vi "Main_UI.vi"(0 "ADC Type":T1, 1 "Edit":bool, 2 "Start":bool, 5 "No. of Bits":u8=1 min=1 max=16, 7 "No. of Channels":u8=1 min=1 max=8, 9 "Sampling Rate(ms)":u8=50 min=50, 11 "Error in":errorcluster, 12 "Confirm":bool, 13 "File Path":path=path "C:/Users/sadhana.suresh/Documents/SVN_Practice/SDLC/Sadhana/SUBMISSION D/Files/Data.txt", 14 "OK Btn":bool) -> (4 "Digital Waveform Graph":digitaldata(graph), 15 "Error out":errorcluster)   [LabVIEW 2020, in "ADC_MultiChannel.lvlib"]
doc: "This the GUI VI. It has a Home page, ADCs Available page and Instructions page. The Instructions are displayed in the Instructions page. The ADCs available with its configuration is displayed in the ADCs Available page. The Home page has all the controls and indicators for the main functionality. Here the ADC can be chosen and its specifications are displayed. When START is pressed the data acquisition starts and the digital data is plotted. Individual channels can be chosen to view them. By pressing EDIT CONFIGURATION the current ADC's specifications can be editted. Panel close will STOP the VI running."
uses:
  ADC_MultiChannel.lvlib
  Typedefs/ADC_Types.ctl
  Typedefs/Queue_Operations.ctl
  Typedefs/Data_Cluster_ip.ctl
  <vilib>/Utility/config.llb/Write Key (I32).vi
  <vilib>/Utility/config.llb/Read Key (I32).vi
  <vilib>/Utility/file.llb/Write Delimited Spreadsheet (I64).vi
  <vilib>/Utility/config.llb/NI_LVConfig.lvlib
panel:
  in  "Tab Control":enum32{"Home", "ADCs Available", "Instructions"}(tab)
  out "Sampling Rate":i32
  out "Channels":i32
  out "Bits":i32
  in  "Channel 1":bool
  in  "Channel 2":bool
  in  "Channel 3":bool
  in  "Channel 4":bool
  in  "Channel 5":bool
  in  "Channel 6":bool
  in  "Channel 7":bool
  in  "Channel 8":bool
  out "Message":string
  in  "Back Btn":bool
  out "Details":string
  out "Instructions":string
  # "ADC"
  # "CHANNEL"
  # "No. of Bits"
  # "No. of Channels"
  # "Sampling Rate"
  # "SELECTOR"
  # "MULTICHANNEL ADC"
  # "SOLITON"
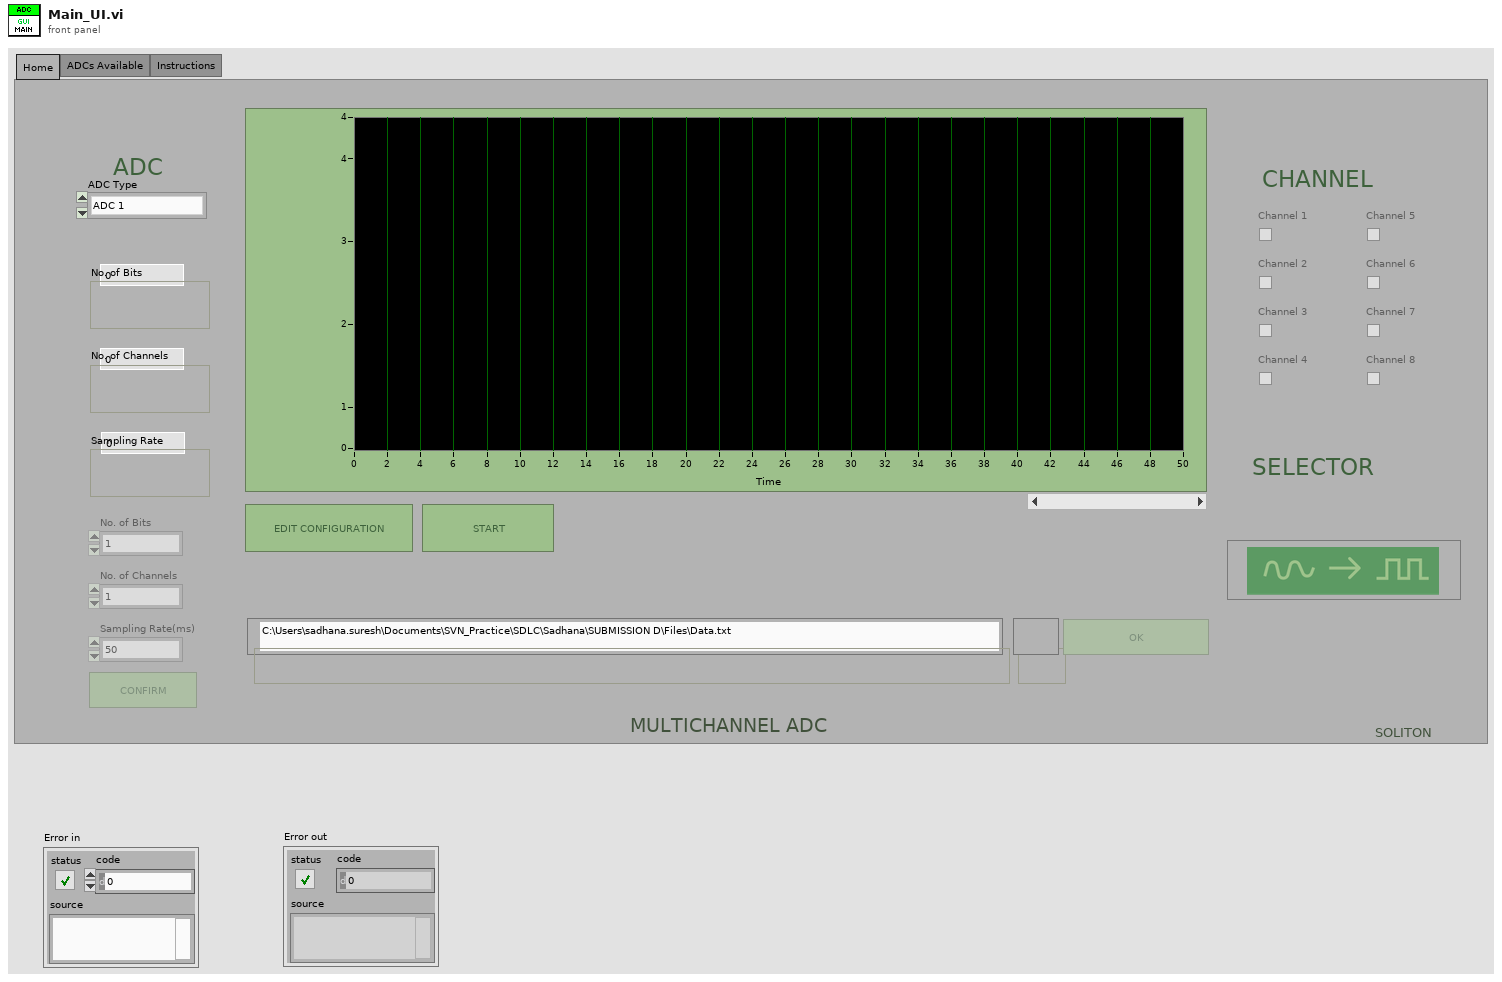
[diagram p1: front panel]
types:
  T1 = typedef "ADC_MultiChannel.lvlib/ADC_Types.ctl" = enum16{"ADC 1", "ADC 2", "ADC 3"}
  T2 = typedef "ADC_MultiChannel.lvlib/Data_Cluster_ip.ctl" = cluster{"ADC Type":string, "Bits":i32, "Channels":i32, "Sampling Rate":i32, "Digital Data":u8[][], "Start":bool, "File Path":path, "Analog Data":dbl[], "Channels ON":bool[], "OK Btn":bool, "Message":string, "Changed Channels":u8, "Changed Bits":u8, "Changed Rate":u8, "ADC Config File":path, "Edit":bool}
  T3 = typedef "ADC_MultiChannel.lvlib/Queue_Operations.ctl" = enum16{"Create Queue", "Enqueue element", "Dequeue", "Flush Queue", "Close Queue"}
  T4 = enum8{"Enabled", "Disabled", "Disabled and Grayed Out"}
  T5 = enum16{"open", "replace", "create", "open or create", "replace or create", "replace or create with confirmation"}
  T6 = typedef "NI_LVConfig.lvlib/Config Data RefNum.ctl" = refnum<k1>
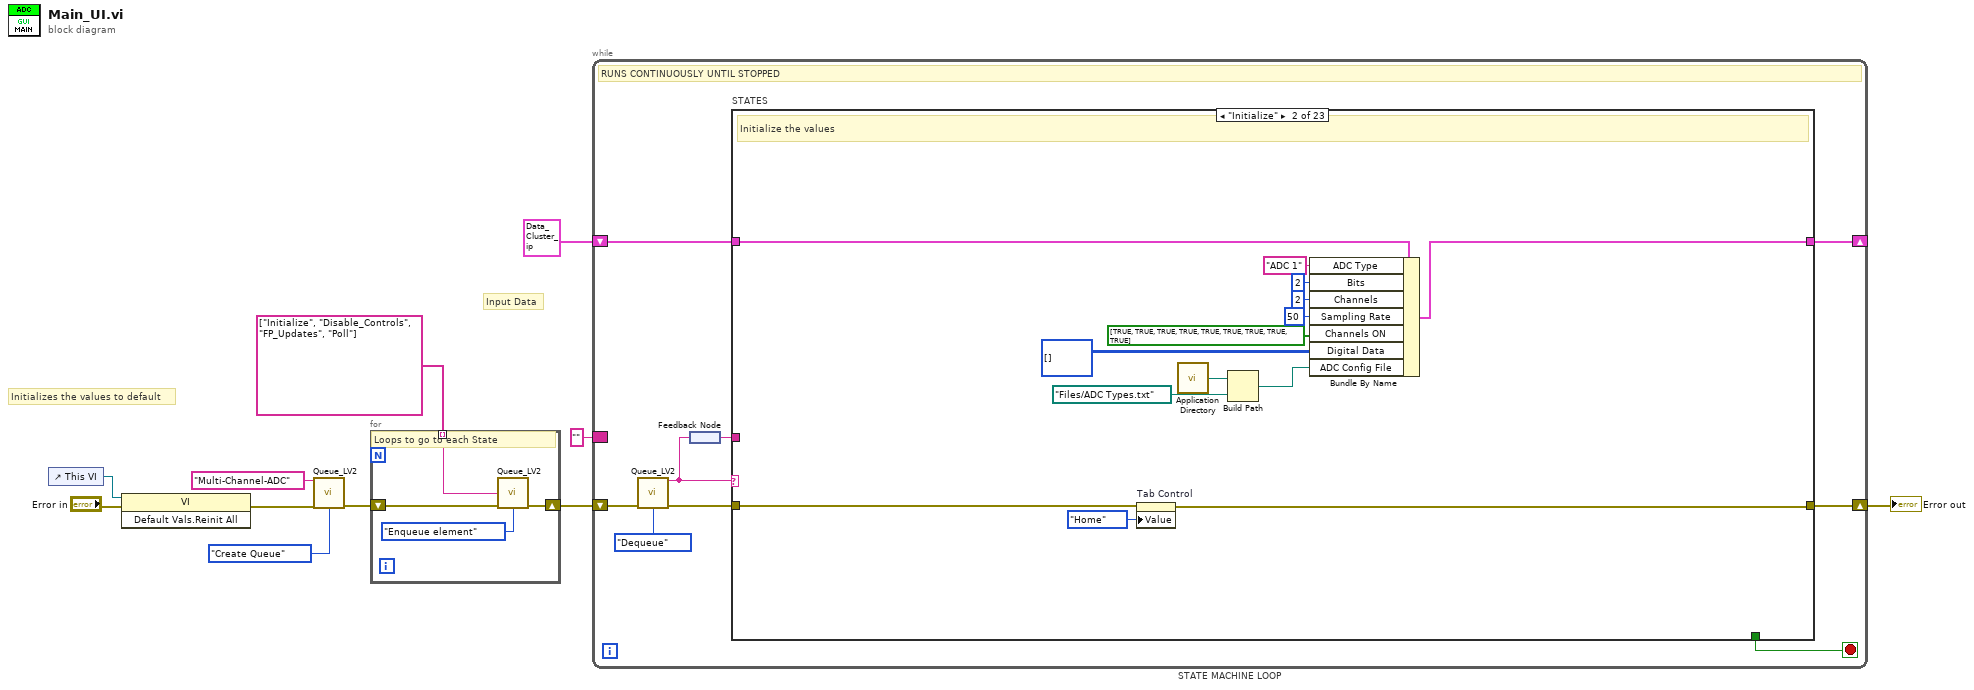
[diagram p0: block diagram]
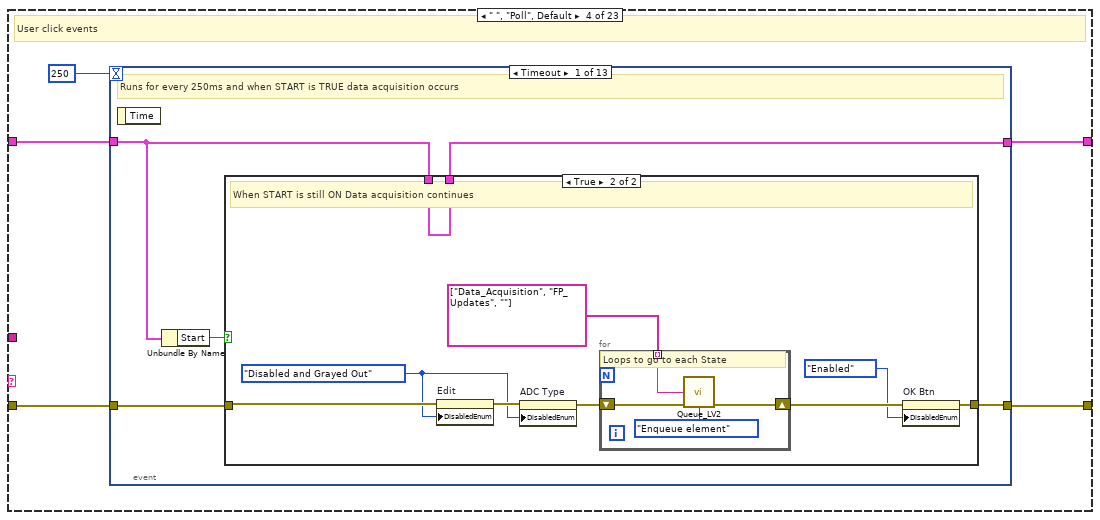
[diagram p4: hidden frame]
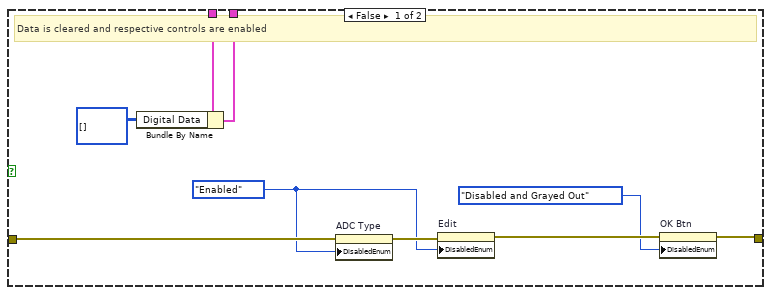
[diagram p5: hidden frame]
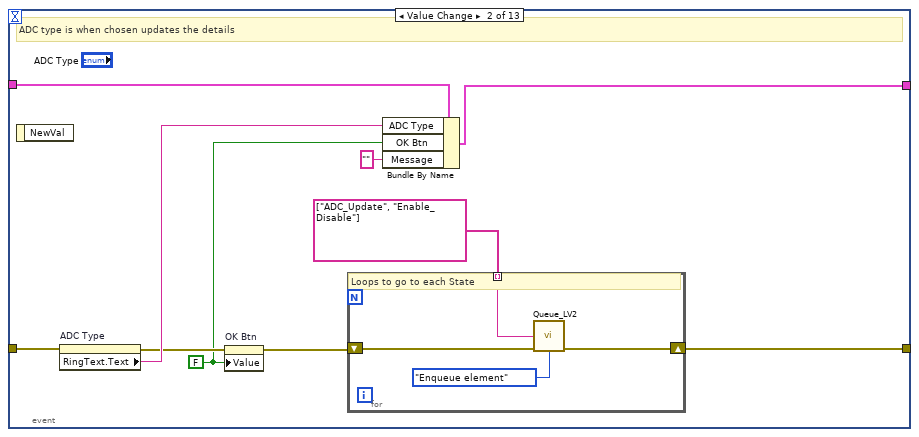
[diagram p6: hidden frame]
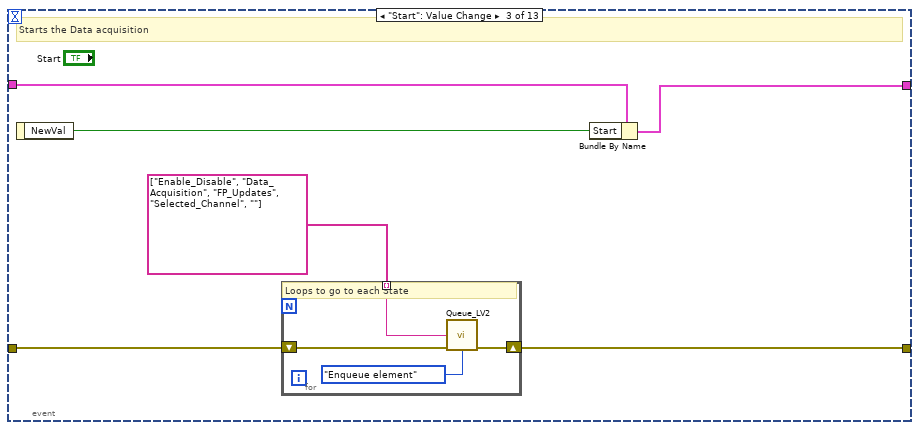
[diagram p7: hidden frame]
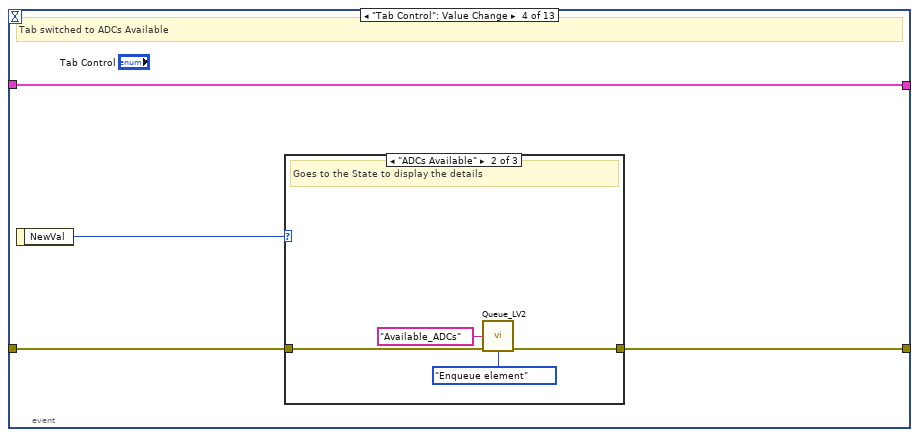
[diagram p8: hidden frame]
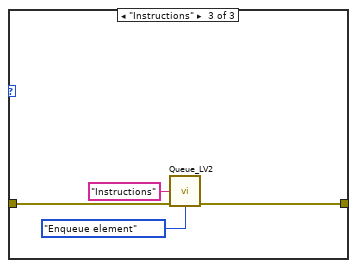
[diagram p10: hidden frame]
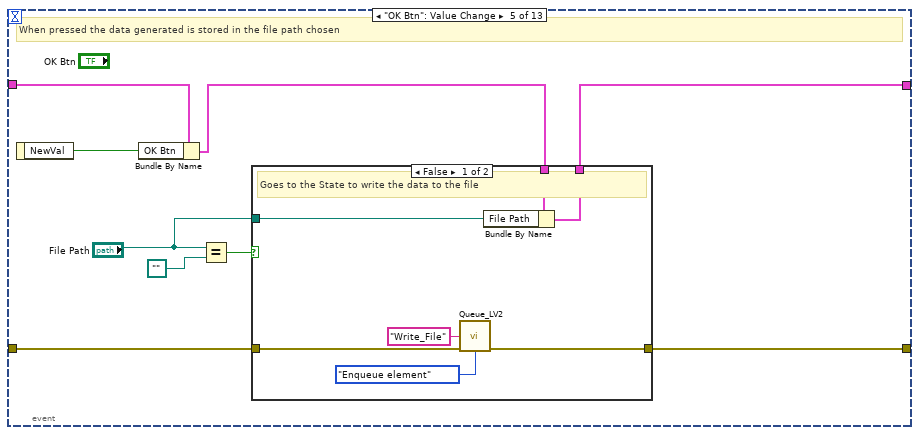
[diagram p11: hidden frame]
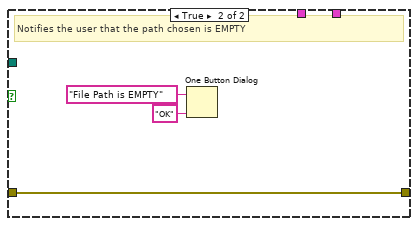
[diagram p12: hidden frame]
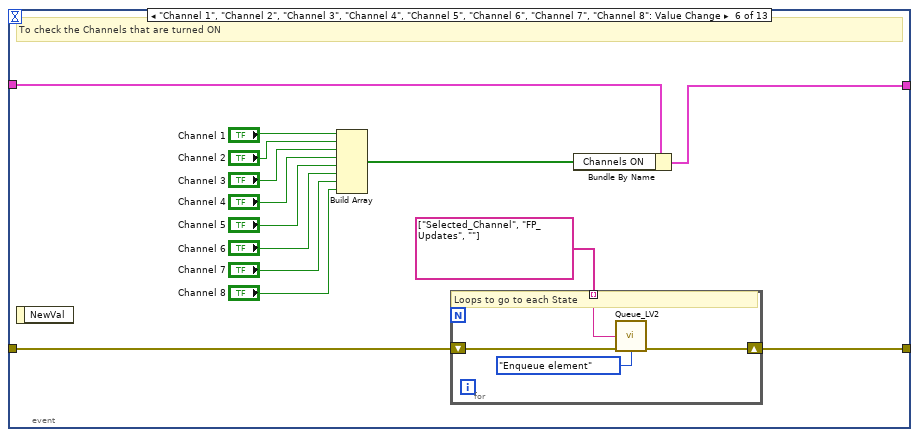
[diagram p13: hidden frame]
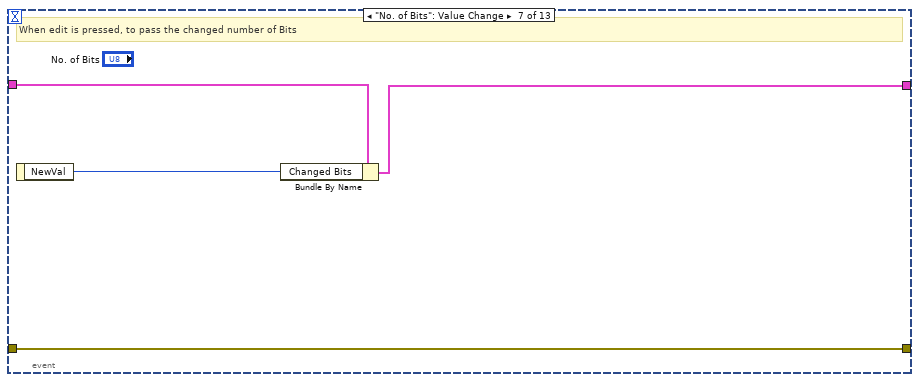
[diagram p14: hidden frame]
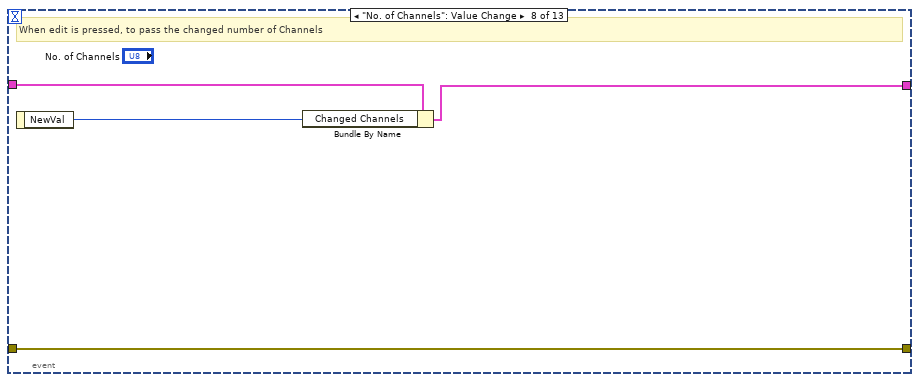
[diagram p15: hidden frame]
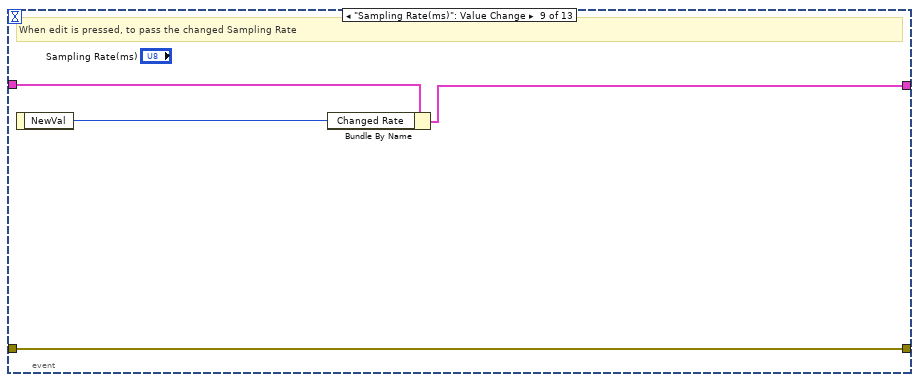
[diagram p16: hidden frame]
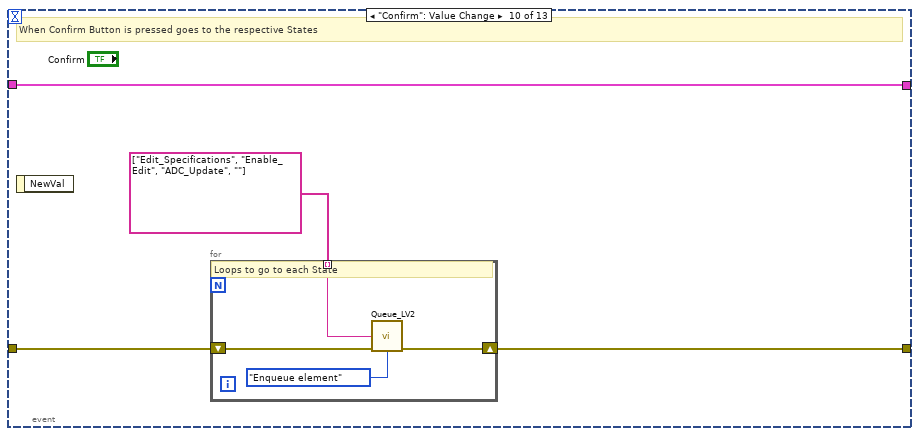
[diagram p17: hidden frame]
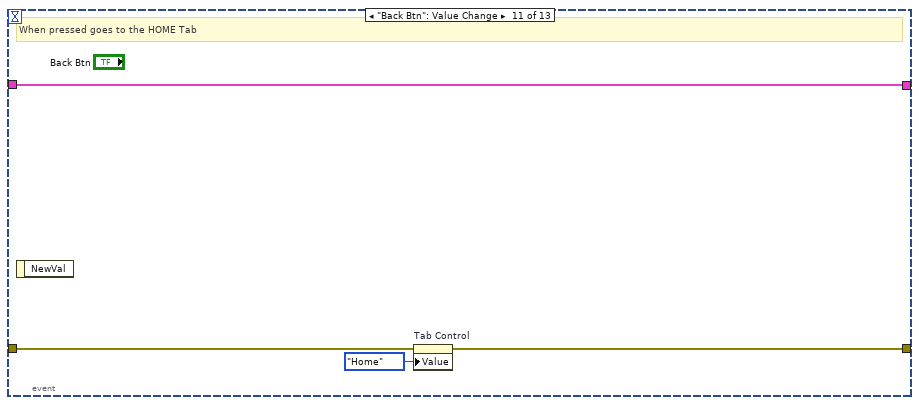
[diagram p18: hidden frame]
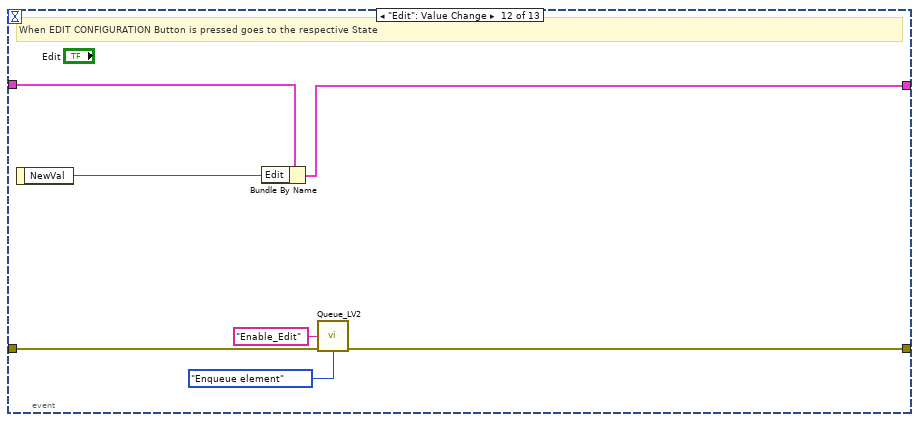
[diagram p19: hidden frame]
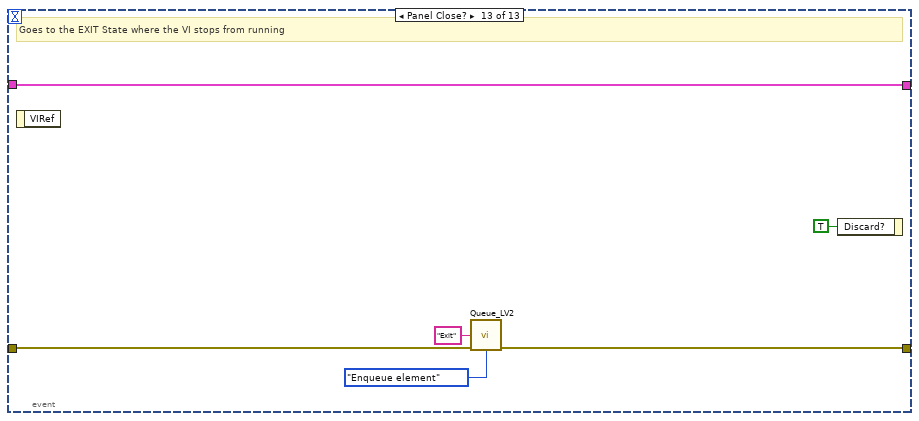
[diagram p20: hidden frame]
diagram:
  # "Input Data"
  # "Initializes the values to default"
  n1 = control-ref of="This VI"() -> (w4:refnum<vi>)
  n2 = invoke class="VI" method="Default Vals.Reinit All"(reference=w4, error in="Error in") -> (error out=w2:errorcluster)  [unwired: 1 in, 2 out]
  n3 = call "Queue_LV2.vi"("Name"="Multi-Channel-ADC", "Error in"=w2, "Queue Operations"=Queue_Operations."Create Queue") -> ("Error out"=w10:errorcluster)  [unwired: 11 in, 1 out]
  n4 = for {
    shift-right: [w14] -> w9
    shift-left: w10 -> [w15]
    tunnel: string[] ["Initialize", "Disable_Controls", "FP_Updates", "Poll"] -> [w12] mode=indexing
    # "Loops to go to each State"
    n5 = call "Queue_LV2.vi"("State"=w12, "Error in"=w15, "Queue Operations"=Queue_Operations."Enqueue element") -> ("Error out"=w14:errorcluster)  [unwired: 11 in, 1 out]
  }
  n6 = while "STATE MACHINE LOOP" {
    shift-right: [w19] -> _
    shift-left: T2 {"ADC Type"="", "Bits"=0, "Channels"=0, "Sampling Rate"=0, "Digital Data"=[], "Start"=FALSE, "File Path"=path "", "Analog Data"=[], "Channels ON"=[], "OK Btn"=FALSE, "Message"="", "Changed Channels"=1, "Changed Bits"=1, "Changed Rate"=50, "ADC Config File"=path "", "Edit"=FALSE} -> [w20]
    shift-right: [w21] -> w6
    shift-left: w9 -> [w24]
    border: "" ("Dequeue State") -> [_]
    stop <- w18 stop-if-true
    # "RUNS CONTINUOUSLY UNTIL STOPPED"
    n7 = call "Queue_LV2.vi"("Error in"=w24, "Queue Operations"=Queue_Operations."Dequeue") -> ("Dequeue State"=w17:string, "Error out"=w22:errorcluster)  [unwired: 12 in]
    n8 = feedback-in #1(w17) -> ()
    n9 = feedback #1() -> (w16:string)
    n10 = case "STATES" shown="\"Initialize\"" w17 {
      tunnel: w22 -> [w25 w28 w41 w44 w187 w191 w205 w344 w361 w363 w372 w399 w412 w439 w454 w489 w496 w503 w516 w520 w526 w529 w543]
      tunnel: [w25 w32 w41 w43 w187 w192 w204 w343 w361 w363 w372 w379 w403 w428 w453 w479 w496 w501 w508 w520 w524 w529 w531] -> w21
      tunnel: w20 -> [w26 w40 w42 w46 w188 w203 w207 w342 w362 w368 w373 w376 w409 w433 w455 w484 w497 w499 w519 w521 w528 w530 w534]
      tunnel: [w26 w35 w42 w45 w188 w203 w207 w342 w362 w368 w373 w375 w408 w426 w455 w482 w497 w499 w519 w521 w528 w530 w534] -> w19
      tunnel: [_ _ _ _ _ _ _ _ _ _ _ _ _ _ _ _ _ _ _ _ TRUE _ _] -> w18
      tunnel: w16 -> [_ _ _ _ _ _ _ _ _ _ _ _ _ _ _ _ _ _ _ _ _ _ w541]
      frame "<---------------------Initialize--------------------->" {
        # "Splitter Case"
      }
      frame "Initialize" {
        # "Initialize the values"
        n11 = property on="Tab Control" class="TabCtl (strict)"(error in=w28, "Value"=enum32{"Home", "ADCs Available", "Instructions"}."Home" ("Tab Control")) -> (error out=w32:errorcluster)  [unwired: 1 in, 1 out]
        n12 = call <vilib>:"Application Directory.vi"() -> ("Application Directory"=w31:path)
        n13 = Build Path(base path=w31, name or relative path=path "Files/ADC Types.txt") -> (appended path=w29:path)
        n14 = Bundle By Name(cluster=w40, "ADC Type"="ADC 1", "Bits"=2, "Channels"=2, "Sampling Rate"=50, "Channels ON"=bool[] [TRUE, TRUE, TRUE, TRUE, TRUE, TRUE, TRUE, TRUE, TRUE], "Digital Data"=u8[][] [], "ADC Config File"=w29) -> (w35:T2)
      }
      frame "<-------------User Click Event--------------->" {
        # "Splitter Case"
      }
      frame " ", "Poll", Default {
        # "User click events"
        n15 = event shown="[0] Timeout" {
          selector: _ -> [_ _ _ _ _ _ _ _ _ _ _ _ _]
          dyn-events: _ -> [_ _ _ _ _ _ _ _ _ _ _ _ _]
          timeout: 250 -> [_ _ _ _ _ _ _ _ _ _ _ _ _]
          tunnel: w46 -> [w49 w84 w91 w102 w114 w137 w151 w157 w161 w165 w173 w176 w186]
          tunnel: [w48 w83 w90 w102 w116 w135 w150 w155 w159 w165 w173 w175 w186] -> w45
          tunnel: w44 -> [w51 w82 w94 w101 w118 w134 w153 w154 w158 w164 w172 w180 w185]
          tunnel: [w50 w76 w93 w100 w117 w133 w153 w154 w158 w163 w171 w179 w184] -> w43
          event Timeout {
            # "Runs for every 250ms and when START is TRUE data acquisition occurs"
            n16 = event-data() -> ()  [unwired: 1 in, 1 out]
            n17 = Unbundle By Name(w49) -> ("Start"=w52:bool)
            n18 = case shown="True" w52 {
              tunnel: w51 -> [w61 w65]
              tunnel: [w54 w63] -> w50
              tunnel: w49 -> [w60 w67]
              tunnel: [w59 w67] -> w48
              frame False {
                w55 = T4."Enabled" ("Disabled")
                # "Data is cleared and respective controls are enabled"
                n19 = Bundle By Name(cluster=w60, "Digital Data"=u8[][] []) -> (w59:T2)
                n20 = property on="ADC Type" class="Enum (strict)"(error in=w61, "DisabledEnum"=w55) -> (error out=w57:errorcluster)  [unwired: 1 in, 1 out]
                n21 = property on="Edit" class="Bool (strict)"(error in=w57, "DisabledEnum"=w55) -> (error out=w56:errorcluster)  [unwired: 1 in, 1 out]
                n22 = property on="OK Btn" class="Bool (strict)"(error in=w56, "DisabledEnum"=T4."Disabled and Grayed Out" ("Disabled")) -> (error out=w54:errorcluster)  [unwired: 1 in, 1 out]
              }
              frame True {
                w64 = T4."Disabled and Grayed Out" ("Disabled")
                # "When START is still ON Data acquisition continues"
                n23 = property on="Edit" class="Bool (strict)"(error in=w65, "DisabledEnum"=w64) -> (error out=w66:errorcluster)  [unwired: 1 in, 1 out]
                n24 = property on="ADC Type" class="Enum (strict)"(error in=w66, "DisabledEnum"=w64) -> (error out=w68:errorcluster)  [unwired: 1 in, 1 out]
                n25 = for {
                  shift-right: [w73] -> w70
                  shift-left: w68 -> [w74]
                  tunnel: string[] ["Data_Acquisition", "FP_Updates", ""] -> [w71] mode=indexing
                  # "Loops to go to each State"
                  n26 = call "Queue_LV2.vi"("State"=w71, "Error in"=w74, "Queue Operations"=Queue_Operations."Enqueue element") -> ("Error out"=w73:errorcluster)  [unwired: 11 in, 1 out]
                }
                n27 = property on="OK Btn" class="Bool (strict)"(error in=w70, "DisabledEnum"=T4."Enabled" ("Disabled")) -> (error out=w63:errorcluster)  [unwired: 1 in, 1 out]
              }
            }
          }
          event Value Change {
            w77 = FALSE ("OK Btn")
            # "ADC type is when chosen updates the details"
            n28 = event-data() -> ()  [unwired: 1 in, 1 out]
            n29 = property on="ADC Type" class="Enum (strict)"(error in=w82) -> (error out=w78:errorcluster, "RingText.Text"=w81:string)  [unwired: 1 in, 1 out]
            n30 = property on="OK Btn" class="Bool (strict)"(error in=w78, "Value"=w77) -> (error out=w79:errorcluster)  [unwired: 1 in, 1 out]
            n31 = for {
              shift-right: [w87] -> w76
              shift-left: w79 -> [w88]
              tunnel: string[] ["ADC_Update", "Enable_Disable"] -> [w85] mode=indexing
              # "Loops to go to each State"
              n32 = call "Queue_LV2.vi"("State"=w85, "Error in"=w88, "Queue Operations"=Queue_Operations."Enqueue element") -> ("Error out"=w87:errorcluster)  [unwired: 11 in, 1 out]
            }
            n33 = Bundle By Name(cluster=w84, "ADC Type"=w81, "OK Btn"=w77, "Message"="") -> (w83:T2)
          }
          event "Start": Value Change {
            # "Starts the Data acquisition"
            n34 = event-data() -> ("NewVal"=w89:bool)  [unwired: 1 in]
            n35 = for {
              shift-right: [w97] -> w93
              shift-left: w94 -> [w98]
              tunnel: string[] ["Enable_Disable", "Data_Acquisition", "FP_Updates", "Selected_Channel", ""] -> [w95] mode=indexing
              # "Loops to go to each State"
              n36 = call "Queue_LV2.vi"("State"=w95, "Error in"=w98, "Queue Operations"=Queue_Operations."Enqueue element") -> ("Error out"=w97:errorcluster)  [unwired: 11 in, 1 out]
            }
            n37 = Bundle By Name(cluster=w91, "Start"=w89) -> (w90:T2)
          }
          event "Tab Control": Value Change {
            # "Tab switched to ADCs Available"
            n38 = event-data() -> ("NewVal"=w99:enum32{"Home", "ADCs Available", "Instructions"})  [unwired: 1 in]
            n39 = case shown="\"ADCs Available\"" w99 {
              tunnel: w101 -> [w103 w106 w111]
              tunnel: [w103 w105 w110] -> w100
              frame "Home", Default {
                # "Nothing Happens"
              }
              frame "ADCs Available" {
                # "Goes to the State to display the details"
                n40 = call "Queue_LV2.vi"("State"="Available_ADCs", "Error in"=w106, "Queue Operations"=Queue_Operations."Enqueue element") -> ("Error out"=w105:errorcluster)  [unwired: 11 in, 1 out]
              }
              frame "Instructions" {
                n41 = call "Queue_LV2.vi"("State"="Instructions", "Error in"=w111, "Queue Operations"=Queue_Operations."Enqueue element") -> ("Error out"=w110:errorcluster)  [unwired: 11 in, 1 out]
              }
            }
          }
          event "OK Btn": Value Change {
            # "When pressed the data generated is stored in the file path chosen"
            n42 = event-data() -> ("NewVal"=w112:bool)  [unwired: 1 in]
            n43 = Bundle By Name(cluster=w114, "OK Btn"=w112) -> (w113:T2)
            n44 = Equal?(x="File Path", y=path "") -> (x = y?=w119:bool)
            n45 = case shown="False" w119 {
              tunnel: w118 -> [w124 w129]
              tunnel: [w123 w129] -> w117
              tunnel: w113 -> [w127 w128]
              tunnel: [w126 w128] -> w116
              tunnel: "File Path" -> [w125 _]
              frame False {
                # "Goes to the State to write the data to the file"
                n46 = call "Queue_LV2.vi"("State"="Write_File", "Error in"=w124, "Queue Operations"=Queue_Operations."Enqueue element") -> ("Error out"=w123:errorcluster)  [unwired: 11 in, 1 out]
                n47 = Bundle By Name(cluster=w127, "File Path"=w125) -> (w126:T2)
              }
              frame True {
                # "Notifies the user that the path chosen is EMPTY"
                n48 = One Button Dialog(message="File Path is EMPTY", button name ("OK")="OK") -> ()  [unwired: 1 out]
              }
            }
          }
          event "Channel 1", "Channel 2", "Channel 3", "Channel 4", "Channel 5", "Channel 6", "Channel 7", "Channel 8": Value Change {
            # "To check the Channels that are turned ON"
            n49 = event-data() -> ()  [unwired: 1 in, 1 out]
            n50 = Build Array("Channel 1", "Channel 2", "Channel 3", "Channel 4", "Channel 5", "Channel 6", "Channel 7", "Channel 8") -> (w136:bool[])
            n51 = for {
              shift-right: [w148] -> w133
              shift-left: w134 -> [w149]
              tunnel: string[] ["Selected_Channel", "FP_Updates", ""] -> [w146] mode=indexing
              # "Loops to go to each State"
              n52 = call "Queue_LV2.vi"("State"=w146, "Error in"=w149, "Queue Operations"=Queue_Operations."Enqueue element") -> ("Error out"=w148:errorcluster)  [unwired: 11 in, 1 out]
            }
            n53 = Bundle By Name(cluster=w137, "Channels ON"=w136) -> (w135:T2)
          }
          event "No. of Bits": Value Change {
            # "When edit is pressed, to pass the changed number of Bits"
            n54 = event-data() -> ("NewVal"=w152:u8)  [unwired: 1 in]
            n55 = Bundle By Name(cluster=w151, "Changed Bits"=w152) -> (w150:T2)
          }
          event "No. of Channels": Value Change {
            # "When edit is pressed, to pass the changed number of Channels"
            n56 = event-data() -> ("NewVal"=w156:u8)  [unwired: 1 in]
            n57 = Bundle By Name(cluster=w157, "Changed Channels"=w156) -> (w155:T2)
          }
          event "Sampling Rate(ms)": Value Change {
            # "When edit is pressed, to pass the changed Sampling Rate"
            n58 = event-data() -> ("NewVal"=w160:u8)  [unwired: 1 in]
            n59 = Bundle By Name(cluster=w161, "Changed Rate"=w160) -> (w159:T2)
          }
          event "Confirm": Value Change {
            # "When Confirm Button is pressed goes to the respective States"
            n60 = event-data() -> ()  [unwired: 1 in, 1 out]
            n61 = for {
              shift-right: [w168] -> w163
              shift-left: w164 -> [w169]
              tunnel: string[] ["Edit_Specifications", "Enable_Edit", "ADC_Update", ""] -> [w166] mode=indexing
              # "Loops to go to each State"
              n62 = call "Queue_LV2.vi"("State"=w166, "Error in"=w169, "Queue Operations"=Queue_Operations."Enqueue element") -> ("Error out"=w168:errorcluster)  [unwired: 11 in, 1 out]
            }
          }
          event "Back Btn": Value Change {
            # "When pressed goes to the HOME Tab"
            n63 = event-data() -> ()  [unwired: 1 in, 1 out]
            n64 = property on="Tab Control" class="TabCtl (strict)"(error in=w172, "Value"=enum32{"Home", "ADCs Available", "Instructions"}."Home" ("Tab Control")) -> (error out=w171:errorcluster)  [unwired: 1 in, 1 out]
          }
          event "Edit": Value Change {
            # "When EDIT CONFIGURATION Button is pressed goes to the respective State"
            n65 = event-data() -> ("NewVal"=w174:bool)  [unwired: 1 in]
            n66 = Bundle By Name(cluster=w176, "Edit"=w174) -> (w175:T2)
            n67 = call "Queue_LV2.vi"("State"="Enable_Edit", "Error in"=w180, "Queue Operations"=Queue_Operations."Enqueue element") -> ("Error out"=w179:errorcluster)  [unwired: 11 in, 1 out]
          }
          event Panel Close? {
            # "Goes to the EXIT State where the VI stops from running"
            n68 = event-data() -> ()  [unwired: 1 in, 1 out]
            n69 = call "Queue_LV2.vi"("State"="Exit", "Error in"=w185, "Queue Operations"=Queue_Operations."Enqueue element") -> ("Error out"=w184:errorcluster)  [unwired: 11 in, 1 out]
            n70 = event-data("Discard?"=TRUE) -> ()  [unwired: 1 in, 1 out]
          }
        }
      }
      frame "<-----------------Enable and Disable---------------->" {
        # "Splitter Case"
      }
      frame "Disable_Controls" {
        w189 = T4."Disabled and Grayed Out" ("Disabled")
        # "Disable the Controls at the time of Initialization"
        n71 = property on="Confirm" class="Bool"(error in=w191, "DisabledEnum"=w189) -> (error out=w190:errorcluster)  [unwired: 1 in, 1 out]
        n72 = property on="Sampling Rate(ms)" class="DigNum (strict)"(error in=w190, "DisabledEnum"=w189) -> (error out=w193:errorcluster)  [unwired: 1 in, 1 out]
        n73 = property on="No. of Bits" class="DigNum (strict)"(error in=w193, "DisabledEnum"=w189) -> (error out=w195:errorcluster)  [unwired: 1 in, 1 out]
        n74 = property on="No. of Channels" class="DigNum (strict)"(error in=w195, "DisabledEnum"=w189) -> (error out=w194:errorcluster)  [unwired: 1 in, 1 out]
        n75 = property on="Channel 1" class="Bool (strict)"(error in=w194, "DisabledEnum"=w189) -> (error out=w202:errorcluster)  [unwired: 1 in, 1 out]
        n76 = property on="Channel 2" class="Bool (strict)"(error in=w202, "DisabledEnum"=w189) -> (error out=w201:errorcluster)  [unwired: 1 in, 1 out]
        n77 = property on="Channel 3" class="Bool (strict)"(error in=w201, "DisabledEnum"=w189) -> (error out=w200:errorcluster)  [unwired: 1 in, 1 out]
        n78 = property on="Channel 4" class="Bool (strict)"(error in=w200, "DisabledEnum"=w189) -> (error out=w199:errorcluster)  [unwired: 1 in, 1 out]
        n79 = property on="Channel 5" class="Bool (strict)"(error in=w199, "DisabledEnum"=w189) -> (error out=w198:errorcluster)  [unwired: 1 in, 1 out]
        n80 = property on="Channel 6" class="Bool (strict)"(error in=w198, "DisabledEnum"=w189) -> (error out=w197:errorcluster)  [unwired: 1 in, 1 out]
        n81 = property on="Channel 7" class="Bool (strict)"(error in=w197, "DisabledEnum"=w189) -> (error out=w196:errorcluster)  [unwired: 1 in, 1 out]
        n82 = property on="Channel 8" class="Bool (strict)"(error in=w196, "DisabledEnum"=w189) -> (error out=w192:errorcluster)  [unwired: 1 in, 1 out]
      }
      frame "Enable_Disable" {
        # "To Enable and Disable Channels according to the number of Channels present"
        n83 = Unbundle By Name(w207) -> ("Channels"=w206:i32)
        n84 = case shown="0, Default" w206 {
          tunnel: w205 -> [w217 w222 w235 w247 w262 w275 w292 w308 w325]
          tunnel: [w209 w221 w234 w246 w261 w276 w291 w309 w326] -> w204
          frame 0, Default {
            w208 = T4."Disabled and Grayed Out" ("Disabled")
            # "All the Channels are disabled"
            n85 = property on="Channel 1" class="Bool (strict)"(error in=w217, "DisabledEnum"=w208) -> (error out=w216:errorcluster)  [unwired: 1 in, 1 out]
            n86 = property on="Channel 2" class="Bool (strict)"(error in=w216, "DisabledEnum"=w208) -> (error out=w215:errorcluster)  [unwired: 1 in, 1 out]
            n87 = property on="Channel 3" class="Bool (strict)"(error in=w215, "DisabledEnum"=w208) -> (error out=w214:errorcluster)  [unwired: 1 in, 1 out]
            n88 = property on="Channel 4" class="Bool (strict)"(error in=w214, "DisabledEnum"=w208) -> (error out=w213:errorcluster)  [unwired: 1 in, 1 out]
            n89 = property on="Channel 5" class="Bool (strict)"(error in=w213, "DisabledEnum"=w208) -> (error out=w212:errorcluster)  [unwired: 1 in, 1 out]
            n90 = property on="Channel 6" class="Bool (strict)"(error in=w212, "DisabledEnum"=w208) -> (error out=w211:errorcluster)  [unwired: 1 in, 1 out]
            n91 = property on="Channel 7" class="Bool (strict)"(error in=w211, "DisabledEnum"=w208) -> (error out=w210:errorcluster)  [unwired: 1 in, 1 out]
            n92 = property on="Channel 8" class="Bool (strict)"(error in=w210, "DisabledEnum"=w208) -> (error out=w209:errorcluster)  [unwired: 1 in, 1 out]
          }
          frame 1 {
            w219 = T4."Disabled and Grayed Out" ("Disabled")
            # "When the total number of Channel is 1 the 1st channel alone is enabled"
            n93 = property on="Channel 1" class="Bool (strict)"(error in=w222, "DisabledEnum"=T4."Enabled" ("Disabled"), "Value"=TRUE ("Channel 1")) -> (error out=w229:errorcluster)  [unwired: 1 in, 1 out]
            n94 = property on="Channel 2" class="Bool (strict)"(error in=w229, "DisabledEnum"=w219) -> (error out=w228:errorcluster)  [unwired: 1 in, 1 out]
            n95 = property on="Channel 3" class="Bool (strict)"(error in=w228, "DisabledEnum"=w219) -> (error out=w227:errorcluster)  [unwired: 1 in, 1 out]
            n96 = property on="Channel 4" class="Bool (strict)"(error in=w227, "DisabledEnum"=w219) -> (error out=w226:errorcluster)  [unwired: 1 in, 1 out]
            n97 = property on="Channel 5" class="Bool (strict)"(error in=w226, "DisabledEnum"=w219) -> (error out=w225:errorcluster)  [unwired: 1 in, 1 out]
            n98 = property on="Channel 6" class="Bool (strict)"(error in=w225, "DisabledEnum"=w219) -> (error out=w224:errorcluster)  [unwired: 1 in, 1 out]
            n99 = property on="Channel 7" class="Bool (strict)"(error in=w224, "DisabledEnum"=w219) -> (error out=w223:errorcluster)  [unwired: 1 in, 1 out]
            n100 = property on="Channel 8" class="Bool (strict)"(error in=w223, "DisabledEnum"=w219) -> (error out=w221:errorcluster)  [unwired: 1 in, 1 out]
          }
          frame 2 {
            w232 = T4."Disabled and Grayed Out" ("Disabled")
            w233 = T4."Enabled" ("Disabled")
            # "When the total number of Channels are 2 the 1st and 2nd channels alone are enabled"
            n101 = property on="Channel 1" class="Bool (strict)"(error in=w235, "DisabledEnum"=w233, "Value"=TRUE ("Channel 1")) -> (error out=w242:errorcluster)  [unwired: 1 in, 1 out]
            n102 = property on="Channel 2" class="Bool (strict)"(error in=w242, "DisabledEnum"=w233, "Value"=TRUE ("Channel 2")) -> (error out=w241:errorcluster)  [unwired: 1 in, 1 out]
            n103 = property on="Channel 3" class="Bool (strict)"(error in=w241, "DisabledEnum"=w232) -> (error out=w240:errorcluster)  [unwired: 1 in, 1 out]
            n104 = property on="Channel 4" class="Bool (strict)"(error in=w240, "DisabledEnum"=w232) -> (error out=w239:errorcluster)  [unwired: 1 in, 1 out]
            n105 = property on="Channel 5" class="Bool (strict)"(error in=w239, "DisabledEnum"=w232) -> (error out=w238:errorcluster)  [unwired: 1 in, 1 out]
            n106 = property on="Channel 6" class="Bool (strict)"(error in=w238, "DisabledEnum"=w232) -> (error out=w237:errorcluster)  [unwired: 1 in, 1 out]
            n107 = property on="Channel 7" class="Bool (strict)"(error in=w237, "DisabledEnum"=w232) -> (error out=w236:errorcluster)  [unwired: 1 in, 1 out]
            n108 = property on="Channel 8" class="Bool (strict)"(error in=w236, "DisabledEnum"=w232) -> (error out=w234:errorcluster)  [unwired: 1 in, 1 out]
          }
          frame 3 {
            w244 = T4."Disabled and Grayed Out" ("Disabled")
            w245 = T4."Enabled" ("Disabled")
            # "When the total number of Channels are 3 the 1st  2nd and 3rd channels alone are enabled"
            n109 = property on="Channel 1" class="Bool (strict)"(error in=w247, "DisabledEnum"=w245, "Value"=TRUE ("Channel 1")) -> (error out=w256:errorcluster)  [unwired: 1 in, 1 out]
            n110 = property on="Channel 2" class="Bool (strict)"(error in=w256, "DisabledEnum"=w245, "Value"=TRUE ("Channel 2")) -> (error out=w255:errorcluster)  [unwired: 1 in, 1 out]
            n111 = property on="Channel 3" class="Bool (strict)"(error in=w255, "DisabledEnum"=w245, "Value"=TRUE ("Channel 3")) -> (error out=w254:errorcluster)  [unwired: 1 in, 1 out]
            n112 = property on="Channel 4" class="Bool (strict)"(error in=w254, "DisabledEnum"=w244) -> (error out=w253:errorcluster)  [unwired: 1 in, 1 out]
            n113 = property on="Channel 5" class="Bool (strict)"(error in=w253, "DisabledEnum"=w244) -> (error out=w252:errorcluster)  [unwired: 1 in, 1 out]
            n114 = property on="Channel 6" class="Bool (strict)"(error in=w252, "DisabledEnum"=w244) -> (error out=w251:errorcluster)  [unwired: 1 in, 1 out]
            n115 = property on="Channel 7" class="Bool (strict)"(error in=w251, "DisabledEnum"=w244) -> (error out=w250:errorcluster)  [unwired: 1 in, 1 out]
            n116 = property on="Channel 8" class="Bool (strict)"(error in=w250, "DisabledEnum"=w244) -> (error out=w246:errorcluster)  [unwired: 1 in, 1 out]
          }
          frame 4 {
            w257 = T4."Disabled and Grayed Out" ("Disabled")
            w258 = T4."Enabled" ("Disabled")
            # "When the total number of Channels are 4 the 1st  2nd  3rd and 4th channels alone are enabled"
            n117 = property on="Channel 1" class="Bool (strict)"(error in=w262, "DisabledEnum"=w258, "Value"=TRUE ("Channel 1")) -> (error out=w271:errorcluster)  [unwired: 1 in, 1 out]
            n118 = property on="Channel 2" class="Bool (strict)"(error in=w271, "DisabledEnum"=w258, "Value"=TRUE ("Channel 2")) -> (error out=w270:errorcluster)  [unwired: 1 in, 1 out]
            n119 = property on="Channel 3" class="Bool (strict)"(error in=w270, "DisabledEnum"=w258, "Value"=TRUE ("Channel 3")) -> (error out=w269:errorcluster)  [unwired: 1 in, 1 out]
            n120 = property on="Channel 4" class="Bool (strict)"(error in=w269, "DisabledEnum"=w258, "Value"=TRUE ("Channel 4")) -> (error out=w268:errorcluster)  [unwired: 1 in, 1 out]
            n121 = property on="Channel 5" class="Bool (strict)"(error in=w268, "DisabledEnum"=w257) -> (error out=w267:errorcluster)  [unwired: 1 in, 1 out]
            n122 = property on="Channel 6" class="Bool (strict)"(error in=w267, "DisabledEnum"=w257) -> (error out=w266:errorcluster)  [unwired: 1 in, 1 out]
            n123 = property on="Channel 7" class="Bool (strict)"(error in=w266, "DisabledEnum"=w257) -> (error out=w265:errorcluster)  [unwired: 1 in, 1 out]
            n124 = property on="Channel 8" class="Bool (strict)"(error in=w265, "DisabledEnum"=w257) -> (error out=w261:errorcluster)  [unwired: 1 in, 1 out]
          }
          frame 5 {
            w272 = T4."Disabled and Grayed Out" ("Disabled")
            w274 = T4."Enabled" ("Disabled")
            # "When the total number of Channels are 5 the 1st  2nd  3rd 4th and 5th channels alone are enabled"
            n125 = property on="Channel 1" class="Bool (strict)"(error in=w275, "DisabledEnum"=w274, "Value"=TRUE ("Channel 1")) -> (error out=w287:errorcluster)  [unwired: 1 in, 1 out]
            n126 = property on="Channel 2" class="Bool (strict)"(error in=w287, "DisabledEnum"=w274, "Value"=TRUE ("Channel 2")) -> (error out=w286:errorcluster)  [unwired: 1 in, 1 out]
            n127 = property on="Channel 3" class="Bool (strict)"(error in=w286, "DisabledEnum"=w274, "Value"=TRUE ("Channel 3")) -> (error out=w285:errorcluster)  [unwired: 1 in, 1 out]
            n128 = property on="Channel 4" class="Bool (strict)"(error in=w285, "DisabledEnum"=w274, "Value"=TRUE ("Channel 4")) -> (error out=w284:errorcluster)  [unwired: 1 in, 1 out]
            n129 = property on="Channel 5" class="Bool (strict)"(error in=w284, "DisabledEnum"=w274, "Value"=TRUE ("Channel 5")) -> (error out=w283:errorcluster)  [unwired: 1 in, 1 out]
            n130 = property on="Channel 6" class="Bool (strict)"(error in=w283, "DisabledEnum"=w272) -> (error out=w282:errorcluster)  [unwired: 1 in, 1 out]
            n131 = property on="Channel 7" class="Bool (strict)"(error in=w282, "DisabledEnum"=w272) -> (error out=w281:errorcluster)  [unwired: 1 in, 1 out]
            n132 = property on="Channel 8" class="Bool (strict)"(error in=w281, "DisabledEnum"=w272) -> (error out=w276:errorcluster)  [unwired: 1 in, 1 out]
          }
          frame 6 {
            w288 = T4."Disabled and Grayed Out" ("Disabled")
            w290 = T4."Enabled" ("Disabled")
            # "When the total number of Channels are 6 the 1st  2nd  3rd 4th  5th and 6th channels alone are enabled"
            n133 = property on="Channel 1" class="Bool (strict)"(error in=w292, "DisabledEnum"=w290, "Value"=TRUE ("Channel 1")) -> (error out=w304:errorcluster)  [unwired: 1 in, 1 out]
            n134 = property on="Channel 2" class="Bool (strict)"(error in=w304, "DisabledEnum"=w290, "Value"=TRUE ("Channel 2")) -> (error out=w303:errorcluster)  [unwired: 1 in, 1 out]
            n135 = property on="Channel 3" class="Bool (strict)"(error in=w303, "DisabledEnum"=w290, "Value"=TRUE ("Channel 3")) -> (error out=w302:errorcluster)  [unwired: 1 in, 1 out]
            n136 = property on="Channel 4" class="Bool (strict)"(error in=w302, "DisabledEnum"=w290, "Value"=TRUE ("Channel 4")) -> (error out=w301:errorcluster)  [unwired: 1 in, 1 out]
            n137 = property on="Channel 5" class="Bool (strict)"(error in=w301, "DisabledEnum"=w290, "Value"=TRUE ("Channel 5")) -> (error out=w300:errorcluster)  [unwired: 1 in, 1 out]
            n138 = property on="Channel 6" class="Bool (strict)"(error in=w300, "DisabledEnum"=w290, "Value"=TRUE ("Channel 6")) -> (error out=w299:errorcluster)  [unwired: 1 in, 1 out]
            n139 = property on="Channel 7" class="Bool (strict)"(error in=w299, "DisabledEnum"=w288) -> (error out=w298:errorcluster)  [unwired: 1 in, 1 out]
            n140 = property on="Channel 8" class="Bool (strict)"(error in=w298, "DisabledEnum"=w288) -> (error out=w291:errorcluster)  [unwired: 1 in, 1 out]
          }
          frame 7 {
            w307 = T4."Enabled" ("Disabled")
            # "When the total number of Channels are 7 the 1st  2nd  3rd 4th  5th  6th and 7th channels alone are enabled"
            n141 = property on="Channel 1" class="Bool (strict)"(error in=w308, "DisabledEnum"=w307, "Value"=TRUE ("Channel 1")) -> (error out=w322:errorcluster)  [unwired: 1 in, 1 out]
            n142 = property on="Channel 2" class="Bool (strict)"(error in=w322, "DisabledEnum"=w307, "Value"=TRUE ("Channel 2")) -> (error out=w321:errorcluster)  [unwired: 1 in, 1 out]
            n143 = property on="Channel 3" class="Bool (strict)"(error in=w321, "DisabledEnum"=w307, "Value"=TRUE ("Channel 3")) -> (error out=w320:errorcluster)  [unwired: 1 in, 1 out]
            n144 = property on="Channel 4" class="Bool (strict)"(error in=w320, "DisabledEnum"=w307, "Value"=TRUE ("Channel 4")) -> (error out=w319:errorcluster)  [unwired: 1 in, 1 out]
            n145 = property on="Channel 5" class="Bool (strict)"(error in=w319, "DisabledEnum"=w307, "Value"=TRUE ("Channel 5")) -> (error out=w318:errorcluster)  [unwired: 1 in, 1 out]
            n146 = property on="Channel 6" class="Bool (strict)"(error in=w318, "DisabledEnum"=w307, "Value"=TRUE ("Channel 6")) -> (error out=w317:errorcluster)  [unwired: 1 in, 1 out]
            n147 = property on="Channel 7" class="Bool (strict)"(error in=w317, "DisabledEnum"=w307, "Value"=TRUE ("Channel 7")) -> (error out=w316:errorcluster)  [unwired: 1 in, 1 out]
            n148 = property on="Channel 8" class="Bool (strict)"(error in=w316, "DisabledEnum"=T4."Disabled and Grayed Out" ("Disabled")) -> (error out=w309:errorcluster)  [unwired: 1 in, 1 out]
          }
          frame 8 {
            w324 = T4."Enabled" ("Disabled")
            # "When the total number of Channels are 8 ALL are enabled"
            n149 = property on="Channel 1" class="Bool (strict)"(error in=w325, "DisabledEnum"=w324, "Value"=TRUE ("Channel 1")) -> (error out=w340:errorcluster)  [unwired: 1 in, 1 out]
            n150 = property on="Channel 2" class="Bool (strict)"(error in=w340, "DisabledEnum"=w324, "Value"=TRUE ("Channel 2")) -> (error out=w339:errorcluster)  [unwired: 1 in, 1 out]
            n151 = property on="Channel 3" class="Bool (strict)"(error in=w339, "DisabledEnum"=w324, "Value"=TRUE ("Channel 3")) -> (error out=w338:errorcluster)  [unwired: 1 in, 1 out]
            n152 = property on="Channel 4" class="Bool (strict)"(error in=w338, "DisabledEnum"=w324, "Value"=TRUE ("Channel 4")) -> (error out=w337:errorcluster)  [unwired: 1 in, 1 out]
            n153 = property on="Channel 5" class="Bool (strict)"(error in=w337, "DisabledEnum"=w324, "Value"=TRUE ("Channel 5")) -> (error out=w336:errorcluster)  [unwired: 1 in, 1 out]
            n154 = property on="Channel 6" class="Bool (strict)"(error in=w336, "DisabledEnum"=w324, "Value"=TRUE ("Channel 6")) -> (error out=w335:errorcluster)  [unwired: 1 in, 1 out]
            n155 = property on="Channel 7" class="Bool (strict)"(error in=w335, "DisabledEnum"=w324, "Value"=TRUE ("Channel 7")) -> (error out=w334:errorcluster)  [unwired: 1 in, 1 out]
            n156 = property on="Channel 8" class="Bool (strict)"(error in=w334, "DisabledEnum"=w324, "Value"=TRUE ("Channel 8")) -> (error out=w326:errorcluster)  [unwired: 1 in, 1 out]
          }
        }
      }
      frame "Enable_Edit" {
        # "This State is performed when the EDIT CONFIGURATION button is pressed where the controls are enabled accordingly"
        n157 = Unbundle By Name(w342) -> ("Edit"=w341:bool)
        n158 = case shown="False" w341 {
          tunnel: w344 -> [w349 w360]
          tunnel: [w346 w354] -> w343
          frame False {
            w347 = T4."Disabled and Grayed Out" ("Disabled")
            # "When EDIT button is OFF  the controls are Disabled"
            n159 = property on="Confirm" class="Bool"(error in=w349, "DisabledEnum"=w347) -> (error out=w348:errorcluster)  [unwired: 1 in, 1 out]
            n160 = property on="No. of Bits" class="DigNum (strict)"(error in=w348, "DisabledEnum"=w347) -> (error out=w351:errorcluster)  [unwired: 1 in, 1 out]
            n161 = property on="No. of Channels" class="DigNum (strict)"(error in=w351, "DisabledEnum"=w347) -> (error out=w352:errorcluster)  [unwired: 1 in, 1 out]
            n162 = property on="Sampling Rate(ms)" class="DigNum (strict)"(error in=w352, "DisabledEnum"=w347) -> (error out=w350:errorcluster)  [unwired: 1 in, 1 out]
            n163 = property on="Start" class="Bool (strict)"(error in=w350, "DisabledEnum"=T4."Enabled" ("Disabled")) -> (error out=w346:errorcluster)  [unwired: 1 in, 1 out]
          }
          frame True {
            w355 = T4."Enabled" ("Disabled")
            # "When EDIT button is ON the controls are Enabled"
            n164 = property on="Confirm" class="Bool"(error in=w360, "DisabledEnum"=w355) -> (error out=w356:errorcluster)  [unwired: 1 in, 1 out]
            n165 = property on="No. of Bits" class="DigNum (strict)"(error in=w356, "DisabledEnum"=w355) -> (error out=w358:errorcluster)  [unwired: 1 in, 1 out]
            n166 = property on="No. of Channels" class="DigNum (strict)"(error in=w358, "DisabledEnum"=w355) -> (error out=w359:errorcluster)  [unwired: 1 in, 1 out]
            n167 = property on="Sampling Rate(ms)" class="DigNum (strict)"(error in=w359, "DisabledEnum"=w355) -> (error out=w357:errorcluster)  [unwired: 1 in, 1 out]
            n168 = property on="Start" class="Bool (strict)"(error in=w357, "DisabledEnum"=T4."Disabled and Grayed Out" ("Disabled")) -> (error out=w354:errorcluster)  [unwired: 1 in, 1 out]
          }
        }
      }
      frame "<--------------Front Panel Updates------------->" {
        # "Splitter Case"
      }
      frame "FP_Updates" {
        # "Updates the Front Panel with the changes"
        n169 = Unbundle By Name(w368) -> ("Bits"=→"Bits":i32, "Channels"=→"Channels":i32, "Sampling Rate"=→"Sampling Rate":i32, "Digital Data"=w367:u8[][], "Message"=→"Message":string)
        n170 = Bundle By Name(cluster=digitaldata {"transitions"=[], "data"=[]} ("waveform"), "data"=w367) -> (→"Digital Waveform Graph":digitaldata)
      }
      frame "<--------------Main Functionalities--------------->" {
        # "Splitter Case"
      }
      frame "Edit_Specifications" {
        # "EDIT button is turned OFF"
        # "Edits the specifications of the available ADCs"
        n171 = Unbundle By Name(w376) -> ("ADC Type"=w388:string, "ADC Config File"=w398:path, "Changed Rate"=w383:u8, "Changed Channels"=w384:u8, "Changed Bits"=w385:u8)
        n172 = property on="Edit" class="Bool (strict)"(error in=w399, "Value"=FALSE ("Edit")) -> (error out=w378:errorcluster)  [unwired: 1 in, 1 out]
        n173 = call <vilib>:"Open Config Data.vi"("error in (no error)"=w378, "configuration file path"=w398) -> ("error out"=w397:errorcluster, "refnum"=w396:T6)  [unwired: 7 in, 1 out]
        n174 = To Long Integer(number=w385) -> (32bit integer=w394:i32)
        n175 = call-poly <vilib>:"Write Key.vi"("section"=w388, "error in (no error)"=w397, "value"=w394, "key"="No of Bits", "refnum"=w396) -> ("error out"=w393:errorcluster, "refnum out"=w390:T6)  [unwired: 4 in, 1 out]
        n176 = To Long Integer(number=w384) -> (32bit integer=w391:i32)
        n177 = call-poly <vilib>:"Write Key.vi"("section"=w388, "error in (no error)"=w393, "value"=w391, "key"="No of Channels", "refnum"=w390) -> ("error out"=w389:errorcluster, "refnum out"=w387:T6)  [unwired: 4 in, 1 out]
        n178 = To Long Integer(number=w383) -> (32bit integer=w382:i32)
        n179 = call-poly <vilib>:"Write Key.vi"("section"=w388, "error in (no error)"=w389, "value"=w382, "key"="Sampling rate", "refnum"=w387) -> ("error out"=w381:errorcluster, "refnum out"=w380:T6)  [unwired: 4 in, 1 out]
        n180 = call <vilib>:"Close Config Data.vi"("error in (no error)"=w381, "refnum"=w380) -> ("error out"=w379:errorcluster)  [unwired: 8 in, 1 out]
        n181 = Bundle By Name(cluster=w376, "Edit"=FALSE) -> (w375:T2)
      }
      frame "ADC_Update" {
        # "Gets the specifications of the ADC chosen from the file"
        n182 = Unbundle By Name(w409) -> ("ADC Type"=w411:string, "ADC Config File"=w400:path)
        n183 = call <vilib>:"Open Config Data.vi"("error in (no error)"=w412, "configuration file path"=w400) -> ("error out"=w410:errorcluster, "refnum"=w402:T6)  [unwired: 7 in, 1 out]
        n184 = call-poly <vilib>:"Read Key.vi"("section"=w411, "error in (no error)"=w410, "key"="No of Bits", "refnum"=w402) -> ("error out"=w413:errorcluster, "value"=w407:i32, "refnum out"=w420:T6)  [unwired: 4 in, 1 out]
        n185 = call-poly <vilib>:"Read Key.vi"("section"=w411, "error in (no error)"=w413, "key"="No of Channels", "refnum"=w420) -> ("error out"=w418:errorcluster, "value"=w406:i32, "refnum out"=w417:T6)  [unwired: 4 in, 1 out]
        n186 = call-poly <vilib>:"Read Key.vi"("section"=w411, "error in (no error)"=w418, "key"="Sampling rate", "refnum"=w417) -> ("error out"=w415:errorcluster, "value"=w405:i32, "refnum out"=w414:T6)  [unwired: 4 in, 1 out]
        n187 = call <vilib>:"Close Config Data.vi"("error in (no error)"=w415, "refnum"=w414) -> ("error out"=w404:errorcluster)  [unwired: 8 in, 1 out]
        n188 = Bundle By Name(cluster=w409, "Bits"=w407, "Channels"=w406, "Sampling Rate"=w405) -> (w408:T2)
        n189 = for {
          shift-right: [w424] -> w403
          shift-left: w404 -> [w425]
          tunnel: string[] ["FP_Updates", "Poll"] -> [w422] mode=indexing
          # "Loops to go to each State"
          n190 = call "Queue_LV2.vi"("State"=w422, "Error in"=w425, "Queue Operations"=Queue_Operations."Enqueue element") -> ("Error out"=w424:errorcluster)  [unwired: 11 in, 1 out]
        }
      }
      frame "Data_Acquisition" {
        # "Data generated and converted to digital is received and processed"
        n191 = Unbundle By Name(w433) -> ("Digital Data"=w434:u8[][], "Bits"=w438:i32, "Channels"=w437:i32, "Sampling Rate"=w436:i32)
        n192 = call "ADC.vi"("Bits"=w438, "Channels"=w437, "Sampling rate"=w436, "Error in"=w439) -> ("Digital 1D"=w435:u8[], "Analog Data"=w431:dbl[], "Error out"=w430:errorcluster)  [unwired: 9 in]
        n193 = Insert Into Array(array=w434, new element=w435) -> (w432:u8[][])  [unwired: 2 in]
        n194 = Bundle By Name(cluster=w433, "Analog Data"=w431, "Digital Data"=w432) -> (w427:T2)
        n195 = Unbundle By Name(w427) -> ("OK Btn"=w429:bool)
        n196 = case shown="True" w429 {
          tunnel: w430 -> [w440 w448]
          tunnel: [w440 w447] -> w428
          tunnel: w427 -> [w443 w444]
          tunnel: [w442 w444] -> w426
          frame False {
            # "When OK btn is FALSE"
            n197 = Bundle By Name(cluster=w443, "Message"="") -> (w442:T2)
          }
          frame True {
            # "When OK btn is TRUE"
            n198 = call "Queue_LV2.vi"("State"="Write_File", "Error in"=w448, "Queue Operations"=Queue_Operations."Enqueue element") -> ("Error out"=w447:errorcluster)  [unwired: 11 in, 1 out]
          }
        }
      }
      frame "Selected_Channel" {
        # "Channel count"
        # "To display the selected Channel"
        n199 = Unbundle By Name(w455) -> ("Channels"=w451:i32, "Bits"=w452:i32, "Channels ON"=w450:bool[])
        n200 = for {
          N: w451 -> [_]
          tunnel: w452 -> [w462]
          shift-right: [w463] -> w453
          shift-left: w454 -> [w464]
          tunnel: w450 -> [w460]
          shift-right: [w458] -> _
          shift-left: 1 ("Numeric") -> [w456]
          # "Index starts from ZERO"
          # "Loops through number of Channels present"
          n201 = Decrement(x=w456) -> (x-1=w457:i32)
          n202 = Index Array(array=w460, index=w457) -> (element=w459:bool)
          n203 = Multiply(x=w456, y=w462) -> (x*y=w461:i32)
          n204 = for {
            N: w462 -> [_]
            shift-right: [w478] -> w463
            shift-left: w464 -> [w475]
            tunnel: w461 -> [w470]
            tunnel: w459 -> [w477]
            tunnel: w456 -> [w468]
            i -> [w466]
            # "Loops through number of Bits"
            n205 = Increment(x=w466) -> (x+1=w465:i32)
            n206 = Subtract(x=w470, y=w465) -> (x-y=w473:i32)
            n207 = Format Into String(format string="%s %d %s %d", error in=w475, "Channel", w468, "Bit" ("input 3"), w465) -> (resulting string=w471:string, error out=w474:errorcluster)  [unwired: 1 in]
            n208 = To Unsigned Long Integer(number=w473) -> (unsigned 32bit integer=w476:u32)
            n209 = property on="Digital Waveform Graph" class="DigitalGraph (strict)"(error in=w474, "Active Plot"=w476, "Plot.Visible?"=w477, "Plot.Plot Name"=w471) -> (error out=w478:errorcluster)  [unwired: 1 in, 1 out]
          }
          n210 = Increment(x=w456) -> (x+1=w458:i32)
        }
      }
      frame "Write_File" {
        # "Writes the digital data to the file chosen"
        n211 = Unbundle By Name(w484) -> ("Digital Data"=w487:u8[][], "File Path"=w488:path)
        n212 = To Quad Integer(1:w487) -> (0:w485:i64[][])
        n213 = Bundle By Name(cluster=w484, "Message"="STORING !!") -> (w482:T2)
        n214 = call-poly <vilib>:"Write Delimited Spreadsheet.vi"("file path (dialog if empty)"=w488, "2D data"=w485, "error in (no error)"=w489, "delimiter (\\t)"="," ("delimiter (\\t)")) -> ("error out"=w481:errorcluster)  [unwired: 10 in, 1 out]
        n215 = Unbundle By Name(w482) -> ("OK Btn"=w480:bool)
        n216 = case shown="False" w480 {
          tunnel: w481 -> [w492 w495]
          tunnel: [w491 w494] -> w479
          frame False {
            # "Enable START button"
            n217 = property on="Start" class="Bool (strict)"(error in=w492, "DisabledEnum"=T4."Enabled" ("Disabled")) -> (error out=w491:errorcluster)  [unwired: 1 in, 1 out]
          }
          frame True {
            # "Disable START button"
            n218 = property on="Start" class="Bool (strict)"(error in=w495, "DisabledEnum"=T4."Disabled and Grayed Out" ("Disabled")) -> (error out=w494:errorcluster)  [unwired: 1 in, 1 out]
          }
        }
      }
      frame "<-------------Read from File and Display-----------> " {
        # "Splitter Case"
      }
      frame "Available_ADCs" {
        # "Displays all the ADC types with its configurations from the txt file"
        n219 = Unbundle By Name(w499) -> ("ADC Config File"=w498:path)
        n220 = Open/Create/Replace File(file path (use dialog)=w498, error in=w503, operation (0:open)=T5."open") -> (refnum out=w507:refnum<file>, error out=w504:errorcluster)  [unwired: 3 in, 1 out]
        n221 = Read from Text File(file (use dialog)=w507, error in=w504) -> (refnum out=w505:refnum<file>, text=→"Details":string, error out=w502:errorcluster)  [unwired: 2 in, 1 out]
        n222 = Close File(refnum=w505, error in=w502) -> (error out=w501:errorcluster)  [unwired: 1 out]
      }
      frame "Instructions" {
        # "Displays the Instructions from the text file"
        n223 = call <vilib>:"Application Directory.vi"() -> ("Application Directory"=w518:path)
        n224 = Build Path(base path=w518, name or relative path=path "Files/Instructions.txt") -> (appended path=w514:path)
        n225 = Open/Create/Replace File(file path (use dialog)=w514, error in=w516, operation (0:open)=T5."open") -> (refnum out=w512:refnum<file>, error out=w513:errorcluster)  [unwired: 3 in, 1 out]
        n226 = Read from Text File(file (use dialog)=w512, error in=w513) -> (refnum out=w509:refnum<file>, text=→"Instructions":string, error out=w510:errorcluster)  [unwired: 2 in, 1 out]
        n227 = Close File(refnum=w509, error in=w510) -> (error out=w508:errorcluster)  [unwired: 1 out]
      }
      frame "<----------------------Exit---------------------->" {
        # "Splitter Case"
      }
      frame "Exit" {
        # "Stops the VI from running"
        n228 = call "Queue_LV2.vi"("Error in"=w526, "Queue Operations"=Queue_Operations."Flush Queue") -> ("Error out"=w525:errorcluster)  [unwired: 12 in, 1 out]
        n229 = call "Queue_LV2.vi"("Error in"=w525, "Queue Operations"=Queue_Operations."Close Queue") -> ("Error out"=w524:errorcluster)  [unwired: 12 in, 1 out]
      }
      frame "<---------------------ERROR-------------------->" {
        # "Splitter Case"
      }
      frame "Error" {
        # "Displays the error if occured"
        n230 = Unbundle By Name(w543) -> ("code"=w540:i32, "source"=w539:string)
        n231 = call <vilib>:"Clear Errors.vi"("error in (no error)"=w543) -> ("error out"=w542:errorcluster)  [unwired: 5 in, 1 out]
        n232 = Format Into String(format string="\nError occurred in State: %s\nError Code: %d\nError Source: %s\n", error in=w542, w541, w540, w539) -> (resulting string=w537:string, error out=w532:errorcluster)  [unwired: 1 in]
        n233 = Two Button Dialog(message=w537, 1:"Abort" ("F button name (\"Cancel\")"), 2:"Continue" ("T button name (\"OK\")")) -> (T button?=w533:bool)
        n234 = case shown="False" w533 {
          tunnel: w532 -> [w547 _]
          tunnel: [w546 errorcluster {"status"=FALSE, "code"=0, "source"=""} ("Error out")] -> w531
          frame False {
            # "Goes to EXIT state"
            n235 = call "Queue_LV2.vi"("State"="Exit", "Error in"=w547, "Queue Operations"=Queue_Operations."Enqueue element") -> ("Error out"=w546:errorcluster)  [unwired: 11 in, 1 out]
          }
          frame True {
            # "Clears the ERROR"
          }
        }
      }
    }
  }
  "Error out" <- w6
